vi "RouterParam.vi"(5 "sysAnalogRx":dbl, 6 "eth":dbl, 7 "rf2Tx":dbl, 8 "error in (no error)":errorcluster caption="错误输入（无错误）", 9 "rf1Tx":dbl, 10 "daOut":dbl, 11 "Path":path) -> (0 "error out":errorcluster caption="错误输出", 3 "router":u8)   [LabVIEW 2015]
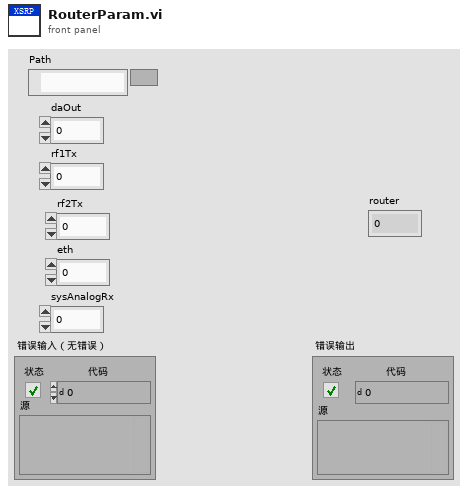
[diagram p1: front panel]
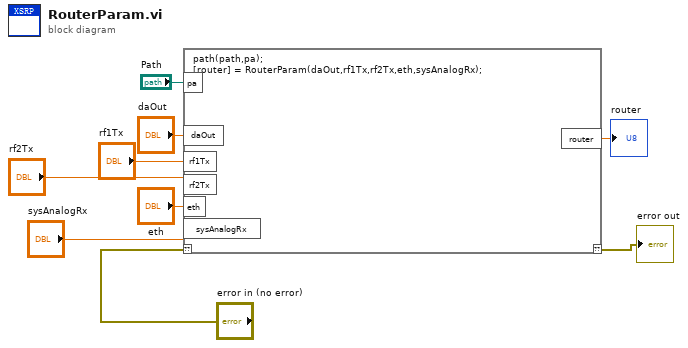
[diagram p0: block diagram]
diagram:
  n1 = script code="path(path,pa);\n[router] = RouterParam(daOut,rf1Tx,rf2Tx,eth,sysAnalogRx);"("??"="error in (no error)", "pa"="Path", "daOut"="daOut", "rf1Tx"="rf1Tx", "rf2Tx"="rf2Tx", "eth"="eth", "sysAnalogRx"="sysAnalogRx") -> ("??"=→"error out":errorcluster, "router"=→"router":dbl)
